vi "Keithley 622x Get NV Settings.vi"(8 "error in":errorcluster, 11 "VISA resource name":refnum<visa-resource-name>) -> (0 "error out":errorcluster, 3 "VISA resource name out":refnum<visa-resource-name>)   [LabVIEW 2021]
uses:
  GPIB/VISA  Send Receive.vi
  Simple VISA Reader/Simple VISA Reader Driver.lvclass
panel:
  out "data string out":string
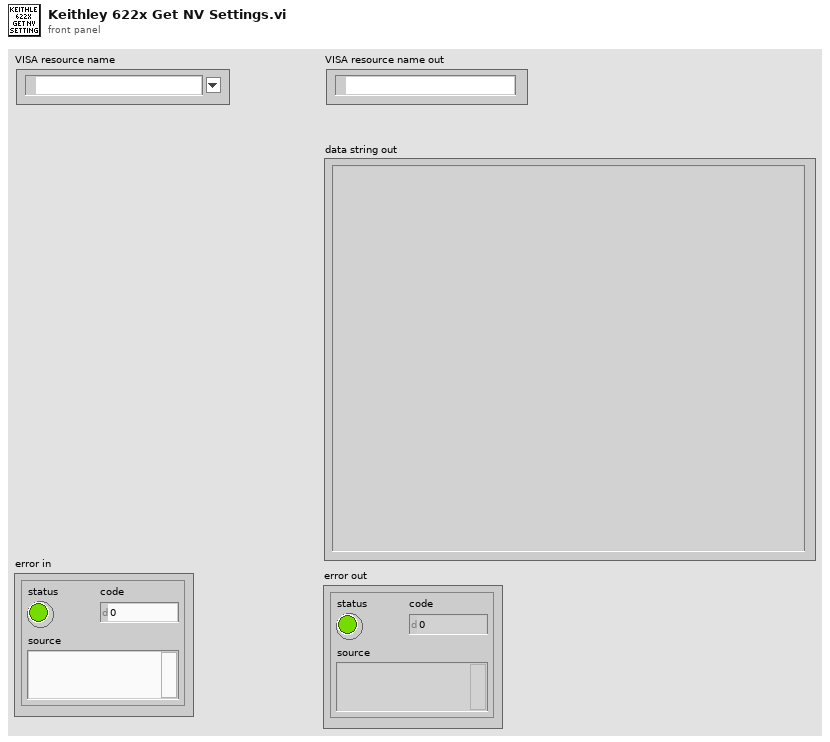
[diagram p1: front panel]
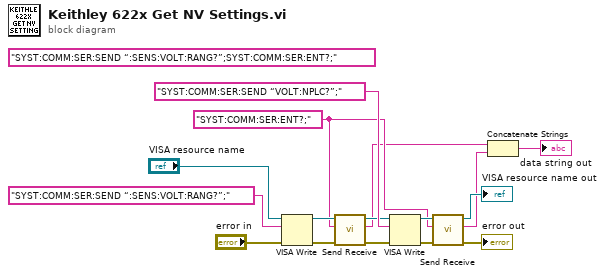
[diagram p0: block diagram]
diagram:
  w5 = "SYST:COMM:SER:ENT?;" ("data string in")
  (unwired) "SYST:COMM:SER:SEND “:SENS:VOLT:RANG?”;SYST:COMM:SER:ENT?;" ("data string in")
  n1 = VISA Write(VISA resource name="VISA resource name", write buffer="SYST:COMM:SER:SEND “:SENS:VOLT:RANG?”;" ("data string in"), error in (no error)="error in") -> (VISA resource name out=w13:refnum<visa-resource-name>, error out=w15:errorcluster)  [unwired: 1 out]
  n2 = call-poly "Send Receive.vi"("error in (no error)"=w15, "data string in"=w5, "VISA Resource Name"=w13) -> ("error out"=w7:errorcluster, "data string out"=w3:string, "VISA Resource Name Out"=w8:refnum<visa-resource-name>)  [unwired: 6 in]
  n3 = VISA Write(VISA resource name=w8, write buffer="SYST:COMM:SER:SEND “VOLT:NPLC?”;" ("data string in"), error in (no error)=w7) -> (VISA resource name out=w10:refnum<visa-resource-name>, error out=w9:errorcluster)  [unwired: 1 out]
  n4 = call-poly "Send Receive.vi"("error in (no error)"=w9, "data string in"=w5, "VISA Resource Name"=w10) -> ("error out"=→"error out":errorcluster, "data string out"=w2:string, "VISA Resource Name Out"=→"VISA resource name out":refnum<visa-resource-name>)  [unwired: 6 in]
  n5 = Concatenate Strings(w3, w2) -> (→"data string out":string)
